vi "main.vi"() -> ()   [LabVIEW 2018]
uses:
  <vilib>/Platform/TimedLoop/XDataNode/timing_clust.ctl
  <vilib>/Platform/TimedLoop/XDataNode/nitl_modes.ctl
  <vilib>/Platform/TimedLoop/XDataNode/wakeup.ctl
  <vilib>/FPGAPlugInAG/myRIO-1900/niLvFpga_Open_myRIO-1900.vi
  <vilib>/rvi/interface/common/dynamic/niFpgaDynamicAddResources.vi
  <vilib>/Utility/error.llb/Error Cluster From Error Code.vi
  <vilib>/rvi/errors/niLvFpgaAdjustHostInterfaceError.vi
  <vilib>/rvi/interface/nirviOpenFPGA/nirviOpenFPGA.xnode
  FPGA Bitfiles/Dentalrobot_FPGATarget_FPGADentalroboto_PTkoih3chUc.lvbitx
  FPGA/FPGA_myRIO.vi
  <vilib>/rvi/interface/nirviReadWriteControl/nirviReadWriteControl.xnode
  <vilib>/Platform/TimedLoop/XDataNode/XDataNode.xnode
  <vilib>/Platform/TimedLoop/XDataNode/XDNodeRunTimeDep.lvlib
  <vilib>/rvi/interface/Simulation/niFpgaSimulationCallBeginRW.vi
  NiFpgaLv.dll
panel:
  in  "Voltage Detect":bool
  in  "temp":i32
  in  "inverse(degree)":i32=90
  in  "limit_mV":u16=2000
  out "Finished Late":dbl
  in  "DIR4":bool
  out "Position4":i32
  in  "Reset 4":bool
  in  "STBY4":bool
  in  "ENA4":bool
  in  "CH4 DC":fxp<+,32,0>
  in  "RPM":string(combo)="150"
  in  "Step":u32 step=200
  in  "Dir":bool=TRUE
  in  "stop":bool
  out "Voltage Detection (mV)":u16(graph)=459
  in  "Inv":bool
  out "mV":u16
  in  "OK Button":bool
  out "position":i32[](array[numeric])
  out "Signal":bool[](array[boolean])
  # "Servor"
  # "Stepper"
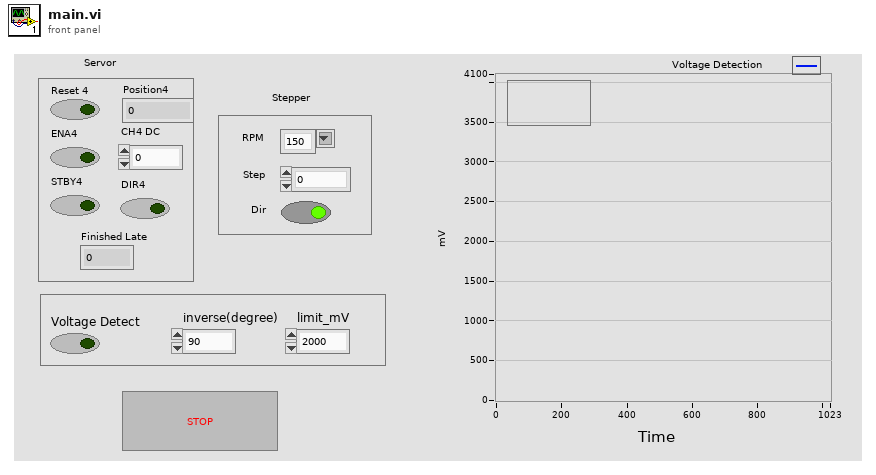
[diagram p1: front panel]
types:
  T1 = typedef "XDNodeRunTimeDep.lvlib/timing_clust.ctl" = cluster{"Expected End [f-1]":u64, "Actual End [f-1]":u64, "Finished Late? [f-1]":bool, "Expected End [i-1]":u64, "Actual End [i-1]":u64, "Finished Late? [i-1]":bool, "Expected Start [i]":u64, "Actual Start [i]":u64, "Expected Start [f]":u64, "Actual Start [f]":u64, "Source Name":string, "Structure Name":string, "Period":i64, "Deadline":i64, "Offset":i64, "Start":i64, "Priority":i32, "Timeout":i32, "Mode":T2, "Wakeup Reason":T3, "Error":errorcluster, "Source Type":string, "Secondary Source Type":string, "Global End Time":u64, "Global Start Time":u64, "Frame Duration":u64, "Iteration Duration":u64, "Assigned CPU":i32, "I/O Scan Engine Mode":u32}
  T2 = typedef "XDNodeRunTimeDep.lvlib/nitl_modes.ctl" = enum32{"No Change", "Process missed periods, maintain original phase", "Discard missed periods, maintain original phase", "Process missed periods, ignore original phase", "Discard missed periods, ignore original phase"}
  T3 = typedef "XDNodeRunTimeDep.lvlib/wakeup.ctl" = enum32{"Normal", "Aborted", "Asynchronous wakeup", "Timing source error", "Timed loop error", "Timeout"}
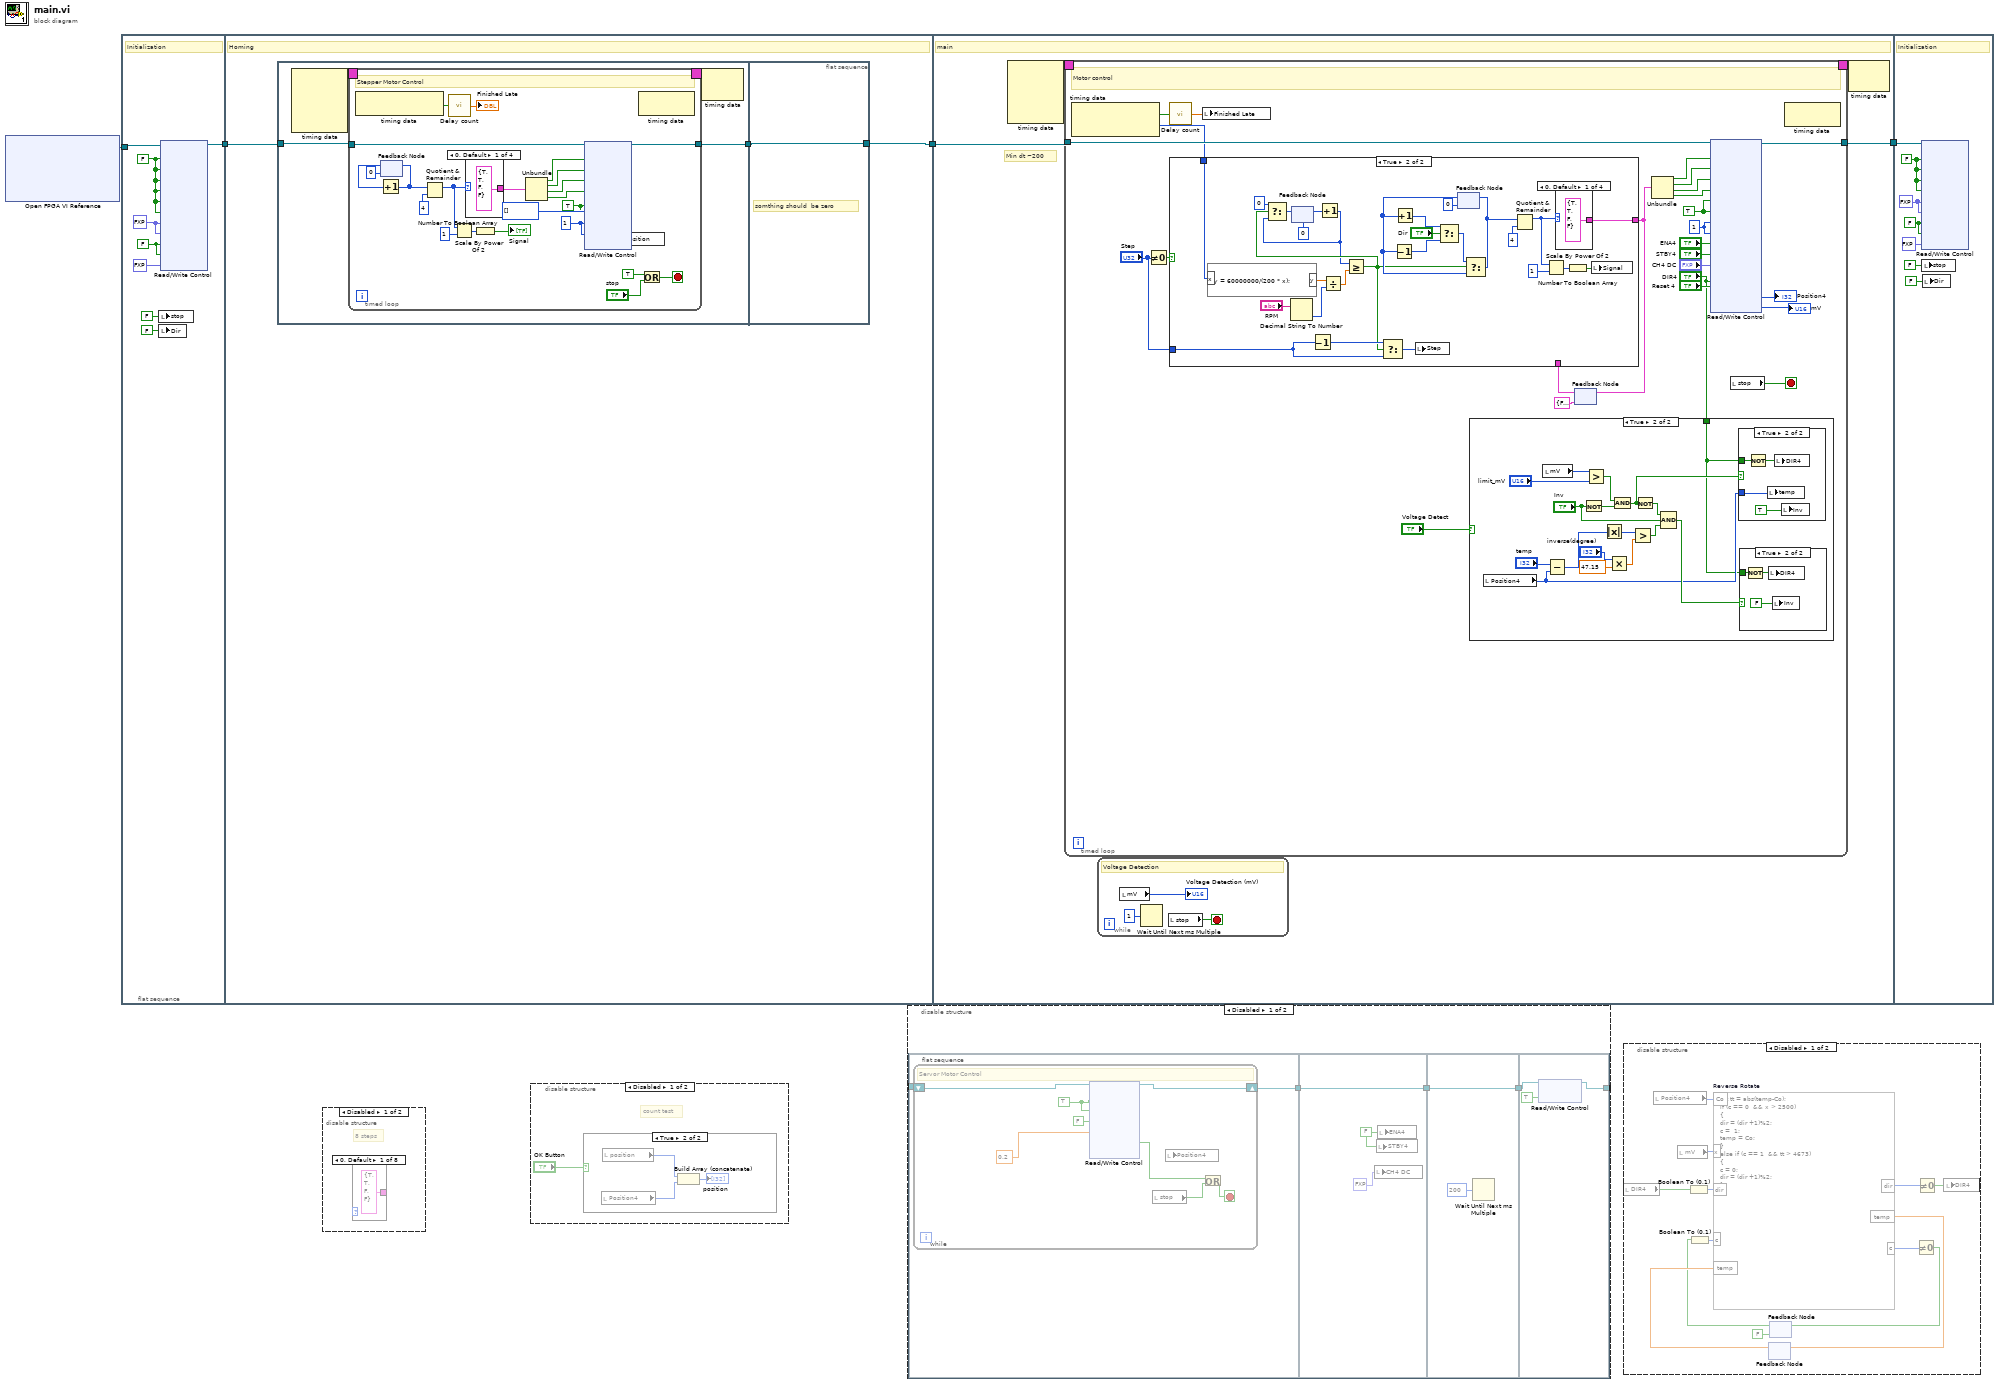
[diagram p0: block diagram]
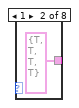
[diagram p6: hidden frame]
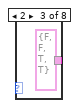
[diagram p7: hidden frame]
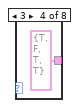
[diagram p8: hidden frame]
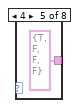
[diagram p9: hidden frame]
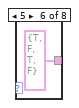
[diagram p10: hidden frame]
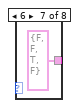
[diagram p11: hidden frame]
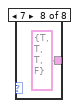
[diagram p12: hidden frame]
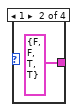
[diagram p14: hidden frame]
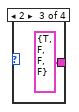
[diagram p15: hidden frame]
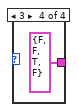
[diagram p16: hidden frame]
diagram:
  n1 = xnode "Open FPGA VI Reference"() -> ("FPGA VI Reference Out"=w1:refnum<k20>)  [unwired: 2 in, 1 out]
  n2 = flat-sequence {
    tunnel: [w11] -> w3
    tunnel: w1 -> [w9]
    tunnel: w3 -> [w14]
    tunnel: [w13] -> w2
    tunnel: [w56] -> w4
    tunnel: w2 -> [w55]
    tunnel: w4 -> [w153]
    frame #0 {
      w8 = FALSE ("ENA4")
      w10 = fxp<+,32,0> 0.0 ("CH1 DC")
      w12 = FALSE ("ENA1")
      # "Initialization"
      n3 = local write "stop"(FALSE ("stop")) -> ()
      n4 = local write "Dir"(FALSE ("Dir")) -> ()
      n5 = xnode "Read/Write Control"("FPGA VI Reference In"=w9, "ENA1"=w12, "STBY1"=w12, "DIR1"=w12, "ENA2"=w12, "STBY2"=w12, "DIR2"=w12, "CH1 DC"=w10, "CH2 DC"=w10, "ENA4"=w8, "STBY4"=w8, "CH4 DC"=fxp<+,32,0> 0.0) -> ("FPGA VI Reference Out"=w11:refnum<k20>)  [unwired: 1 in, 1 out]
    }
    frame #1 {
      # "Homing"
      n6 = flat-sequence {
        tunnel: [w17] -> w15
        tunnel: w14 -> [w16]
        tunnel: w15 -> [w52]
        tunnel: [w52] -> w13
        frame #0 {
          n7 = node-c288() -> (w20:T1)  [unwired: 4 in]
          n8 = timed-loop {
            timing: w20 -> [_]
            timing-out: [_] -> w19
            tunnel: w16 -> [w28]
            tunnel: [w27] -> w17
            stop <- w26 stop-if-true
            w41 = 1 ("CH1 DC")
            w42 = TRUE ("STBY1")
            # "Stepper Motor Control"
            n9 = node-c288() -> (w29:bool)  [unwired: 1 in]
            n10 = feedback #1(0) -> (w38:i32)
            n11 = Increment(x=w38) -> (x+1=w30:i32)
            n12 = feedback-in #1(w30) -> ()
            n13 = Quotient & Remainder(x=w30, y=4) -> (x-y*floor(x/y)=w24:i32)  [unwired: 1 out]
            n14 = call "Delay count.vi"("Finished Late? [i-1]"=w29) -> ("Count"=→"Finished Late":dbl)
            n15 = Scale By Power Of 2(n=w24, x=u32 1) -> (x*2^n=w36:u32)
            n16 = case shown="0, Default" w24 {
              tunnel: [cluster{bool, bool, bool, bool} {TRUE, TRUE, FALSE, FALSE} cluster{bool, bool, bool, bool} {FALSE, FALSE, TRUE, TRUE} cluster{bool, bool, bool, bool} {TRUE, FALSE, FALSE, FALSE} cluster{bool, bool, bool, bool} {FALSE, FALSE, TRUE, FALSE}] -> w35
              frame 0, Default {
              }
              frame 1 {
              }
              frame 2 {
              }
              frame 3 {
              }
            }
            n17 = Number To Boolean Array(number=w36) -> (Boolean array=→"Signal":bool[])
            n18 = Unbundle(w35) -> (w34:bool, w33:bool, w32:bool, w31:bool)
            n19 = xnode "Read/Write Control"("FPGA VI Reference In"=w28, "ENA1"=w34, "DIR1"=w33, "ENA2"=w32, "DIR2"=w31, "STBY1"=w42, "STBY2"=w42, "CH1 DC"=w41, "CH2 DC"=w41) -> ("FPGA VI Reference Out"=w27:refnum<k20>)  [unwired: 1 in, 2 out]
            n20 = node-c288() -> ()  [unwired: 1 in, 1 out]
            n21 = Or(x=TRUE, y="stop") -> (x .or. y?=w26:bool)
          }
          n22 = local write "position"(i32[] []) -> ()
          n23 = node-c288(w19) -> ()  [unwired: 1 out]
        }
        frame #1 {
          # "somthing should  be zero"
        }
      }
    }
    frame #2 {
      # "Min dt ~200"
      # "main"
      n24 = node-c288() -> (w54:T1)  [unwired: 4 in]
      n25 = timed-loop {
        timing: w54 -> [_]
        timing-out: [_] -> w53
        tunnel: [w84] -> w56
        tunnel: w55 -> [w83]
        stop <- w68 stop-if-true
        w77 = 1 ("CH1 DC")
        w81 = TRUE ("STBY1")
        # "Motor control"
        n26 = node-c288() -> (w66:bool, w67:i64)  [unwired: 1 in]
        n27 = Not Equal To 0?(x="Step") -> (x != 0?=w76:bool)
        n28 = call "Delay count.vi"("Finished Late? [i-1]"=w66) -> ("Count"=w65:dbl)
        n29 = local write "Finished Late"(w65) -> ()
        n30 = case shown="True" "Voltage Detect" {
          tunnel: "DIR4" -> [_ w88]
          frame False {
          }
          frame True {
            n31 = local read "Position4"() -> (w90:i32)
            n32 = local read "mV"() -> (w92:u16)
            n33 = Subtract(x="temp", y=w90) -> (x-y=w96:i32)
            n34 = Not(x="Inv") -> (.not. x?=w100:bool)
            n35 = Greater?(x=w92, y="limit_mV") -> (0:w101:bool)
            n36 = Absolute Value(x=w96) -> (abs(x)=w97:i32)
            n37 = Multiply(x="inverse(degree)", y=47.15) -> (x*y=w85:dbl)
            n38 = And(x=w101, y=w100) -> (x .and. y?=w93:bool)
            n39 = Greater?(x=w97, y=w85) -> (0:w98:bool)
            n40 = Not(x=w93) -> (.not. x?=w99:bool)
            n41 = Compound Arithmetic op=AND(w99, "Inv", w98) -> (w94:bool)
            n42 = case shown="True" w93 {
              tunnel: w88 -> [_ w108]
              tunnel: w90 -> [_ w107]
              frame False {
              }
              frame True {
                n43 = Not(x=w108) -> (.not. x?=w106:bool)
                n44 = local write "temp"(w107) -> ()
                n45 = local write "DIR4"(w106) -> ()
                n46 = local write "Inv"(TRUE ("Inv")) -> ()
              }
            }
            n47 = case shown="True" w94 {
              tunnel: w88 -> [_ w104]
              frame False {
              }
              frame True {
                n48 = Not(x=w104) -> (.not. x?=w103:bool)
                n49 = local write "DIR4"(w103) -> ()
                n50 = local write "Inv"(FALSE ("Inv")) -> ()
              }
            }
          }
        }
        n51 = feedback #2(cluster{bool, bool, bool, bool} {FALSE, FALSE, FALSE, FALSE}) -> (w74:cluster{bool, bool, bool, bool})
        n52 = case shown="True" w76 {
          tunnel: [w109 w136] -> w69
          tunnel: "Step" -> [_ w128]
          tunnel: w74 -> [w109 _]
          tunnel: w67 -> [_ w111]
          frame False {
          }
          frame True {
            # "convert  dt to rpm"
            n53 = formula code="y = 60000000/(200 * x);"("x"=w111) -> ("y"=w110:dbl)
            n54 = Decimal String To Number(string="RPM") -> (number=w112:i32)  [unwired: 2 in, 1 out]
            n55 = feedback #3(0) -> (w122:i32)
            n56 = Decrement(x=w128) -> (x-1=w127:u32)
            n57 = Increment(x=w122) -> (x+1=w121:i32)
            n58 = Divide(x=w110, y=w112) -> (x/y=w115:dbl)
            n59 = Greater Or Equal?(x=w121, y=w115) -> (x >= y?=w125:bool)
            n60 = Select(t=0, s=w125, f=w121) -> (s? t:f=w123:i32)
            n61 = feedback-in #3(w123) -> ()
            n62 = Select(t=w127, s=w125, f=w128) -> (s? t:f=w129:u32)
            n63 = local write "Step"(w129) -> ()
            n64 = feedback #4(0) -> (w131:i32)
            n65 = Decrement(x=w131) -> (x-1=w130:i32)
            n66 = Increment(x=w131) -> (x+1=w132:i32)
            n67 = Select(t=w132, s="Dir", f=w130) -> (s? t:f=w126:i32)
            n68 = Select(t=w126, s=w125, f=w131) -> (s? t:f=w118:i32)
            n69 = feedback-in #4(w118) -> ()
            n70 = Quotient & Remainder(x=w118, y=4) -> (x-y*floor(x/y)=w114:i32)  [unwired: 1 out]
            n71 = Scale By Power Of 2(n=w114, x=u32 1) -> (x*2^n=w116:u32)
            n72 = case shown="0, Default" w114 {
              tunnel: [cluster{bool, bool, bool, bool} {TRUE, TRUE, FALSE, FALSE} cluster{bool, bool, bool, bool} {FALSE, FALSE, TRUE, TRUE} cluster{bool, bool, bool, bool} {TRUE, FALSE, FALSE, FALSE} cluster{bool, bool, bool, bool} {FALSE, FALSE, TRUE, FALSE}] -> w136
              frame 0, Default {
              }
              frame 1 {
              }
              frame 2 {
              }
              frame 3 {
              }
            }
            n73 = Number To Boolean Array(number=w116) -> (Boolean array=w113:bool[])
            n74 = local write "Signal"(w113) -> ()
          }
        }
        n75 = feedback-in #2(w69) -> ()
        n76 = Unbundle(w69) -> (w82:bool, w80:bool, w79:bool, w78:bool)
        n77 = xnode "Read/Write Control"("FPGA VI Reference In"=w83, "ENA1"=w82, "DIR1"=w80, "ENA2"=w79, "DIR2"=w78, "STBY1"=w81, "STBY2"=w81, "CH1 DC"=w77, "CH2 DC"=w77, "ENA4"="ENA4", "STBY4"="STBY4", "CH4 DC"="CH4 DC", "DIR4"="DIR4", "Reset 4"="Reset 4") -> ("FPGA VI Reference Out"=w84:refnum<k20>, "Position4"=→"Position4":i32, "Channel4"=→"mV":u16)  [unwired: 1 in, 1 out]
        n78 = local read "stop"() -> (w68:bool)
        n79 = node-c288() -> ()  [unwired: 1 in, 1 out]
      }
      n80 = while {
        stop <- w59 stop-if-true
        # "Voltage Detection"
        n81 = local read "mV"() -> (→"Voltage Detection (mV)":u16)
        n82 = Wait Until Next ms Multiple(millisecond multiple=u32 1) -> ()  [unwired: 1 out]
        n83 = local read "stop"() -> (w59:bool)
      }
      n84 = node-c288(w53) -> ()  [unwired: 1 out]
    }
    frame #3 {
      w150 = FALSE ("ENA4")
      w151 = fxp<+,32,0> 0.0 ("CH1 DC")
      w152 = FALSE ("ENA1")
      # "Initialization"
      n85 = xnode "Read/Write Control"("FPGA VI Reference In"=w153, "ENA1"=w152, "STBY1"=w152, "ENA2"=w152, "STBY2"=w152, "CH1 DC"=w151, "CH2 DC"=w151, "ENA4"=w150, "STBY4"=w150, "CH4 DC"=fxp<+,32,0> 0.0) -> ()  [unwired: 1 in, 2 out]
      n86 = local write "stop"(FALSE ("stop")) -> ()
      n87 = local write "Dir"(FALSE ("Dir")) -> ()
    }
  }
  n88 = disable-structure shown="Disabled" {
    frame Disabled {
      # "8 steps"
      n89 = case shown="0, Default" {
        selector: _ -> [_ _ w157 _ _ _ _ _]
        tunnel: [cluster{bool, bool, bool, bool} {TRUE, TRUE, FALSE, FALSE} cluster{bool, bool, bool, bool} {TRUE, TRUE, TRUE, TRUE} cluster{bool, bool, bool, bool} {FALSE, FALSE, TRUE, TRUE} cluster{bool, bool, bool, bool} {TRUE, FALSE, TRUE, TRUE} cluster{bool, bool, bool, bool} {TRUE, FALSE, FALSE, FALSE} cluster{bool, bool, bool, bool} {TRUE, FALSE, TRUE, FALSE} cluster{bool, bool, bool, bool} {FALSE, FALSE, TRUE, FALSE} cluster{bool, bool, bool, bool} {TRUE, TRUE, TRUE, FALSE}] -> _
        frame 0, Default {
        }
        frame 1 {
        }
        frame 2 {
        }
        frame 3 {
        }
        frame 4 {
        }
        frame 5 {
        }
        frame 6 {
        }
        frame 7 {
        }
      }
    }
    frame Enabled {
    }
  }
  n90 = disable-structure shown="Disabled" {
    frame Disabled {
      # "count test"
      n91 = case shown="True" "OK Button" {
        frame False {
        }
        frame True {
          n92 = local read "Position4"() -> (w165:i32)
          n93 = local read "position"() -> (w166:i32[])
          n94 = Build Array (concatenate)(w166, w165) -> (→"position":i32[])
        }
      }
    }
    frame Enabled {
    }
  }
  n95 = disable-structure shown="Disabled" {
    disable-tunnel: [w167 _] -> _
    frame Disabled {
      n96 = flat-sequence {
        tunnel: _ -> [w172]
        tunnel: [w171] -> w170
        tunnel: w170 -> [w184]
        tunnel: [w184] -> w169
        tunnel: w169 -> [w186]
        tunnel: [w186] -> w168
        tunnel: [w187] -> w167
        tunnel: w168 -> [w189]
        frame #0 {
          n97 = while {
            shift-right: [w180] -> w171
            shift-left: w172 -> [w181]
            stop <- w177 stop-if-true
            w179 = TRUE ("ENA4")
            # "Servor Motor Control"
            n98 = xnode "Read/Write Control"("FPGA VI Reference In"=w181, "ENA4"=w179, "STBY4"=w179, "DIR4"=FALSE, "CH4 DC"=0.2) -> ("FPGA VI Reference Out"=w180:refnum<k20>, "C1"=w173:bool, "Position4"=w174:i32)  [unwired: 1 in, 1 out]
            n99 = local read "stop"() -> (w175:bool)
            n100 = local read "Position4"() -> ()  [unwired: 1 in]
            n101 = Or(x=w173, y=w175) -> (x .or. y?=w177:bool)
          }
        }
        frame #1 {
          w183 = FALSE ("ENA4")
          n102 = local write "CH4 DC"(fxp<+,32,0> 0.0 ("CH4 DC")) -> ()
          n103 = local write "STBY4"(w183) -> ()
          n104 = local write "ENA4"(w183) -> ()
        }
        frame #2 {
          n105 = Wait Until Next ms Multiple(millisecond multiple=u32 200) -> ()  [unwired: 1 out]
        }
        frame #3 {
          n106 = xnode "Read/Write Control"("FPGA VI Reference In"=w189, "Reset 4"=TRUE) -> ("FPGA VI Reference Out"=w187:refnum<k20>)  [unwired: 1 in, 1 out]
        }
      }
    }
    frame Enabled {
    }
  }
  n107 = disable-structure shown="Disabled" {
    frame Disabled {
      n108 = local read "DIR4"() -> (w202:bool)
      n109 = local read "Position4"() -> (w200:i32)
      n110 = local read "mV"() -> (w199:u16)
      n111 = Boolean To (0,1)(Boolean=w202) -> (0, 1=w190:i16)
      n112 = feedback #5() -> (w198:dbl)  [unwired: 1 in]
      n113 = feedback #6(FALSE) -> (w195:bool)
      n114 = Boolean To (0,1)(Boolean=w195) -> (0, 1=w193:i16)
      n115 = formula code="int tt = abs(temp-Co);\nif (c == 0  && x > 2500)\n{\ndir = (dir +1)%2;\nc =  1;\ntemp = Co;\n}\nelse if (c == 1  && tt > 4673)\n{\nc = 0;\ndir = (dir +1)%2;\n}" "Reverse Rotate"("x"=w199, "dir"=w190, "c"=w193, "Co"=w200, "temp"=w198) -> ("dir"=w191:i16, "c"=w192:i16, "temp"=w197:dbl)
      n116 = feedback-in #5(w197) -> ()
      n117 = Not Equal To 0?(x=w192) -> (x != 0?=w194:bool)
      n118 = feedback-in #6(w194) -> ()
      n119 = Not Equal To 0?(x=w191) -> (x != 0?=w201:bool)
      n120 = local write "DIR4"(w201) -> ()
    }
    frame Enabled {
    }
  }
